vi "resetEditArrayButtons.vi"(9 "editpos":i32, 10 "editArray":T1[](array[typedef])) -> (2 "editOut":T1[](array[typedef]))   [LabVIEW 2014]
uses:
  typeDefs/editControl.ctl
  typeDefs/variantFlat.ctl
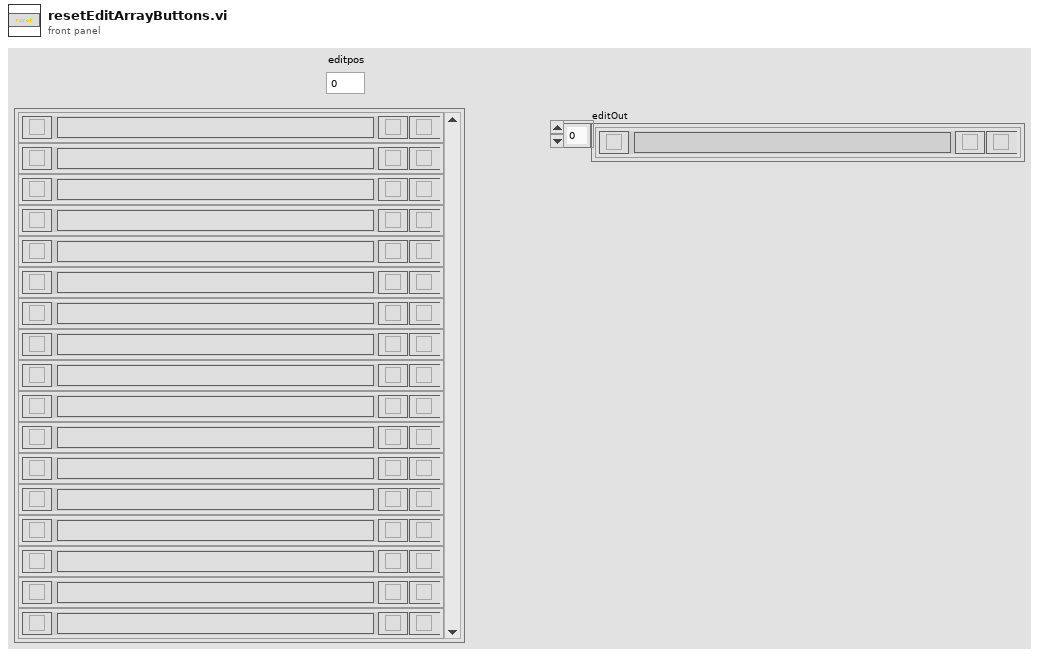
[diagram p1: front panel]
types:
  T1 = typedef "editControl.ctl" = cluster{"edit":bool, "info":string, "variantFlat":T2, "codeCluster":cluster{"code":u8[][]}, "del":bool, "ins":bool}
  T2 = typedef "variantFlat.ctl" = cluster{"type string":i16[], "data string":string}
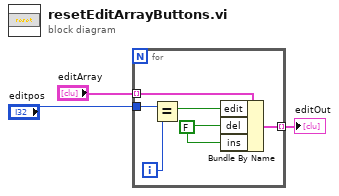
[diagram p0: block diagram]
diagram:
  n1 = for {
    tunnel: "editArray" -> [w9] mode=indexing
    tunnel: [w7] -> w2 mode=indexing
    tunnel: "editpos" -> [w6]
    i -> [w5]
    w8 = FALSE ("edit")
    n2 = Equal?(x=w6, y=w5) -> (x = y?=w4:bool)
    n3 = Bundle By Name(cluster=w9, "edit"=w4, "del"=w8, "ins"=w8) -> (w7:T1)
  }
  "editOut" <- w2
